vi "Settings Dialog.vi"(8 "error in (no error)":errorcluster, 11 "Settings in":T1) -> (0 "error out":errorcluster, 1 "Cancelled?":bool, 2 "UI Refresh Needed?":bool, 3 "Settings out":T1)   [LabVIEW 2018, in "Settings.lvlib"]
doc: "Dialog for selecting user specified settings."
uses:
  Settings.lvlib
  Settings.ctl
  Acquisition/Hardware Configuration.ctl
  Acquisition/Signal Type.ctl
  Logging/Logging Configuration.ctl
  TypeDef/Error LED.ctl
  <vilib>/Utility/xml.llb/Write to XML File(string).vi
  Acquisition/Acquisition.lvlib
  Logging/Logging.lvlib
panel:
  in  "Log File Path":path
  in  "Cancel Button":bool
  in  "OK Button":bool
  # "Non visible portion of dialog (needed for connector pane)."
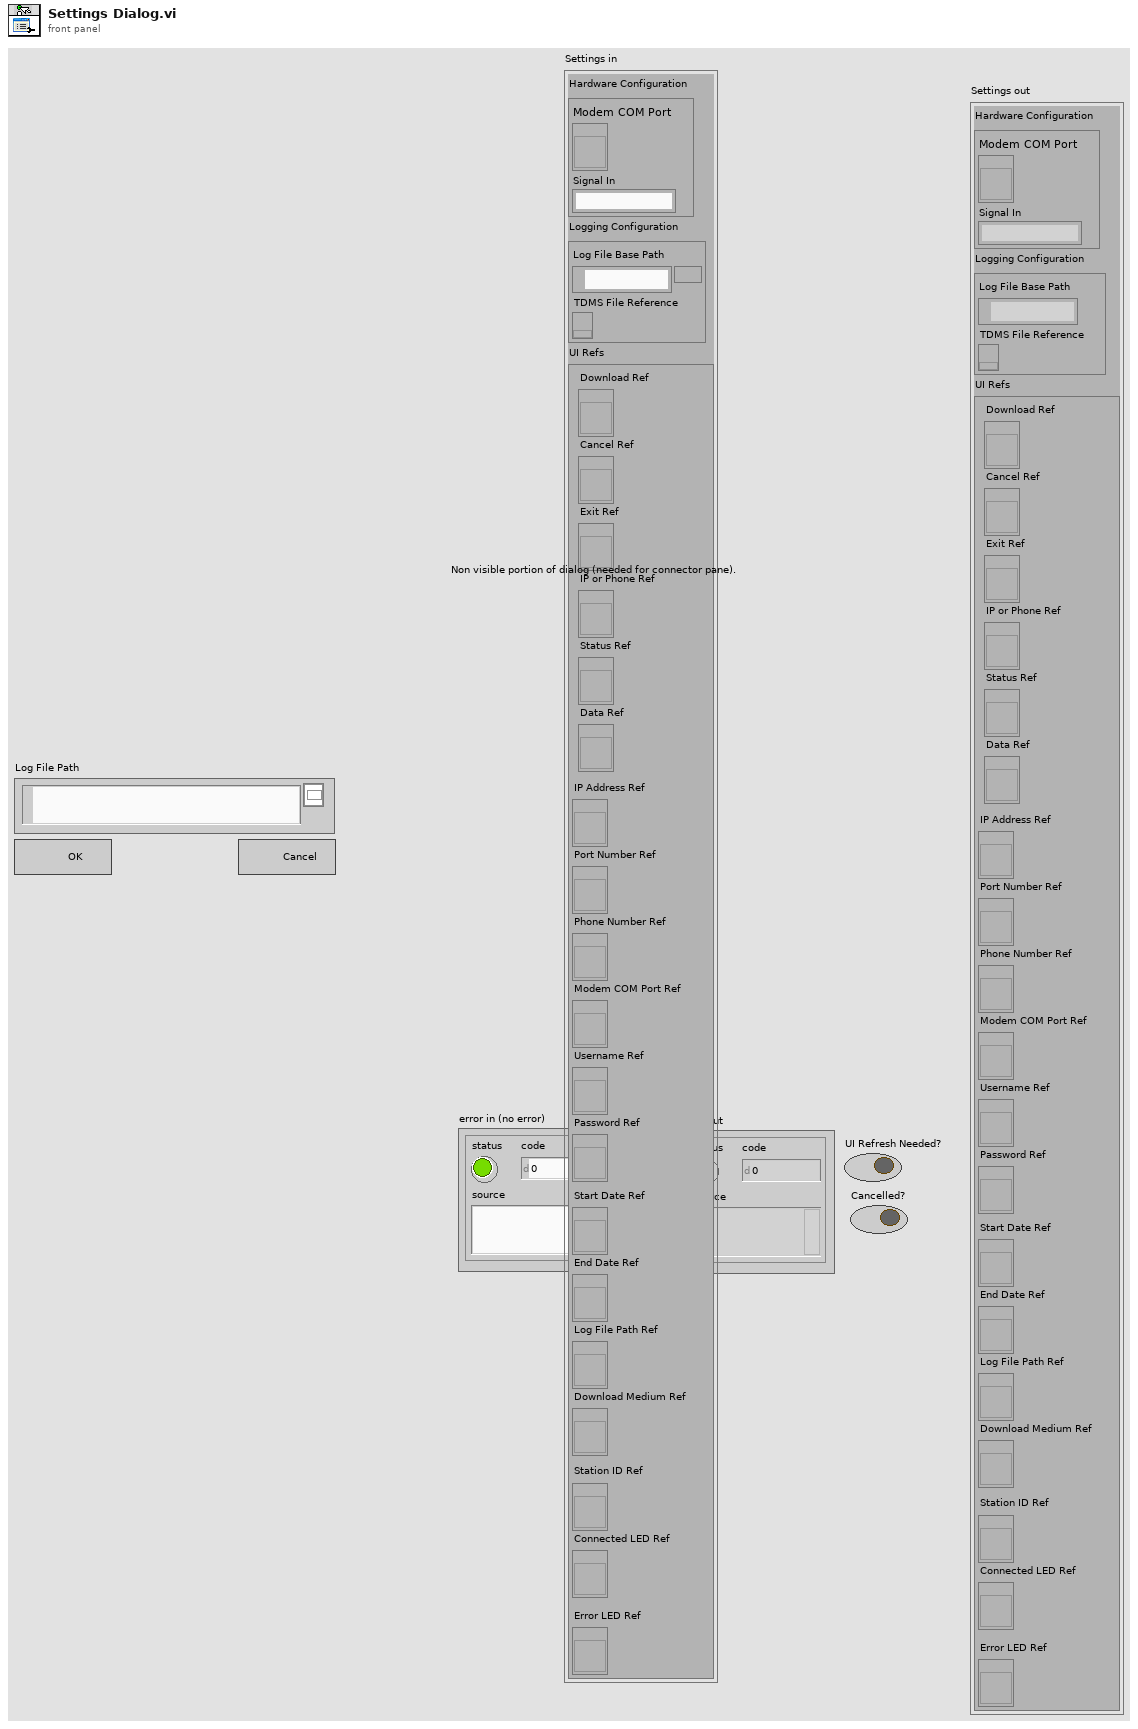
[diagram p1: front panel]
types:
  T1 = typedef "Settings.lvlib/Settings.ctl" = cluster{"Hardware Configuration":T2, "Logging Configuration":T4, "UI Refs":cluster{"Download Ref":refnum<vi>, "Cancel Ref":refnum<vi>, "Exit Ref":refnum<vi>, "IP or Phone Ref":refnum<vi>, "Status Ref":refnum<vi>, "Data Ref":refnum<vi>, "IP Address Ref":refnum<vi>, "Port Number Ref":refnum<vi>, "Phone Number Ref":refnum<vi>, "Modem COM Port Ref":refnum<vi>, "Username Ref":refnum<vi>, "Password Ref":refnum<vi>, "Start Date Ref":refnum<vi>, "End Date Ref":refnum<vi>, "Log File Path Ref":refnum<vi>, "Download Medium Ref":refnum<vi>, "Station ID Ref":refnum<vi>, "Connected LED Ref":refnum<vi>, "Error LED Ref":refnum<vi>}}
  T2 = typedef "Acquisition.lvlib/Hardware Configuration.ctl" = cluster{"Modem COM Port":refnum<vi>, "Signal In":T3}
  T3 = typedef "Acquisition.lvlib/Signal Type.ctl" = string
  T4 = typedef "Logging.lvlib/Logging Configuration.ctl" = cluster{"Log File Base Path":path, "TDMS File Reference":refnum<k34>}
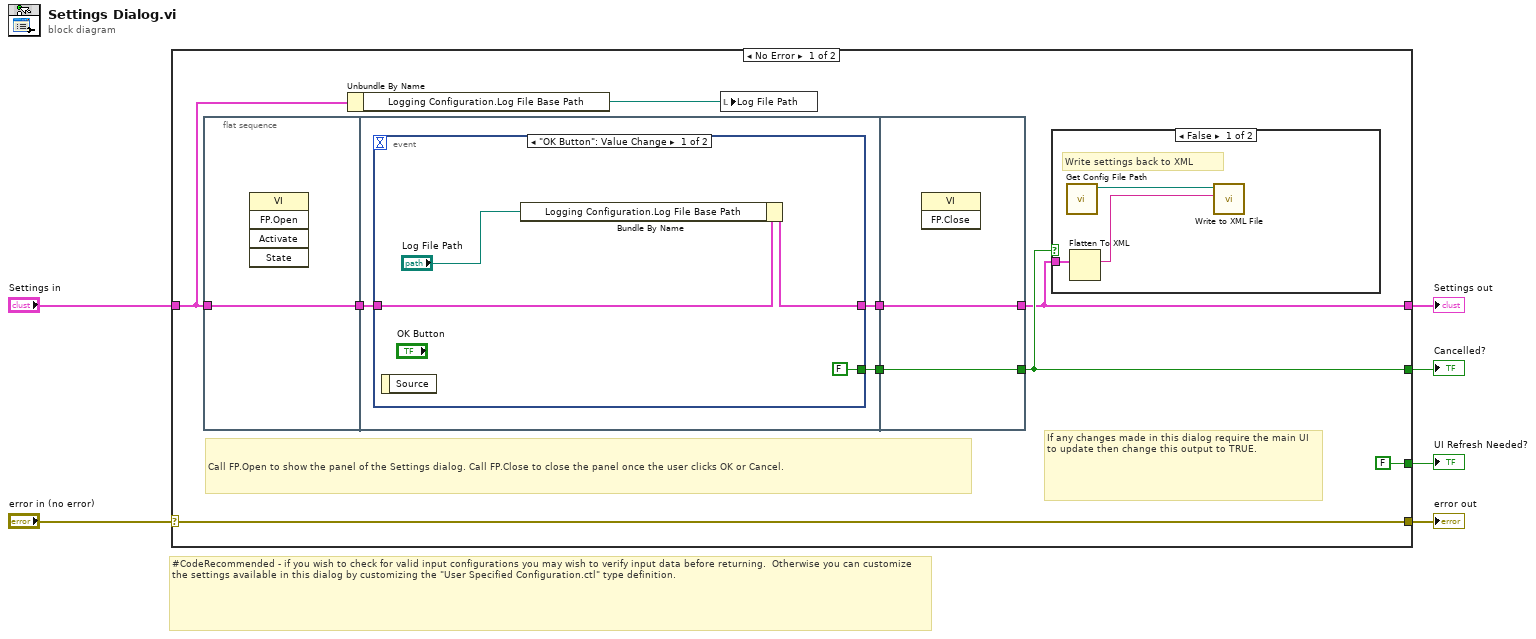
[diagram p0: block diagram]
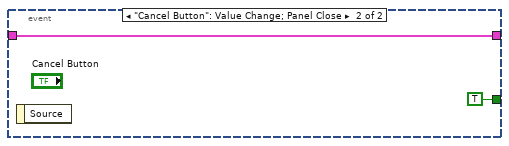
[diagram p2: hidden frame]
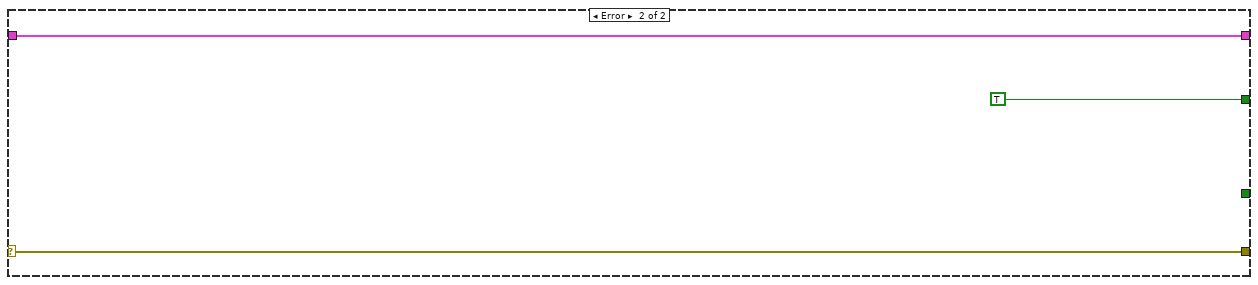
[diagram p4: hidden frame]
diagram:
  # "#CodeRecommended - if you wish to check for valid input configurations you may wish to verify input data before returning.  Otherwise you can customize the settings available in this dialog by customizing the \"User Specified Configuration.ctl\" type definition."
  n1 = case shown="No Error" "error in (no error)" {
    selector: "error in (no error)" -> [w15 w33]
    tunnel: [w15 w33] -> w5
    tunnel: "Settings in" -> [w11 w32]
    tunnel: [w12 w32] -> w3
    tunnel: [FALSE ("UI Refresh Needed?") _] -> w2
    tunnel: [w13 TRUE ("UI Refresh Needed?")] -> w1
    frame No Error {
      # "Call FP.Open to show the panel of the Settings dialog. Call FP.Close to close the panel once the user clicks OK or Cancel."
      # "If any changes made in this dialog require the main UI to update then change this output to TRUE."
      n2 = flat-sequence {
        tunnel: w11 -> [w16]
        tunnel: [w16] -> w9
        tunnel: w9 -> [w17]
        tunnel: [w19] -> w8
        tunnel: [w18] -> w7
        tunnel: [w26] -> w12
        tunnel: [w27] -> w13
        tunnel: w8 -> [w27]
        tunnel: w7 -> [w26]
        frame #0 {
          n3 = invoke class="VI" method="FP.Open"() -> ()  [unwired: 5 in, 5 out]
        }
        frame #1 {
          n4 = event shown="[0] \"OK Button\": Value Change" {
            selector: _ -> [_ _]
            dyn-events: _ -> [_ _]
            timeout: _ -> [_ _]
            tunnel: [w21 w25] -> w18
            tunnel: w17 -> [w22 w25]
            tunnel: [FALSE ("UI Refresh Needed?") TRUE ("UI Refresh Needed?")] -> w19
            event "OK Button": Value Change {
              n5 = event-data() -> ()  [unwired: 1 in, 1 out]
              n6 = Bundle By Name(cluster=w22, "Logging Configuration.Log File Base Path"="Log File Path") -> (w21:T1)
            }
            event "Cancel Button": Value Change; Panel Close {
              n7 = event-data() -> ()  [unwired: 1 in, 1 out]
            }
          }
        }
        frame #2 {
          n8 = invoke class="VI" method="FP.Close"() -> ()  [unwired: 3 in, 3 out]
        }
      }
      n9 = Unbundle By Name(w11) -> ("Logging Configuration.Log File Base Path"=w10:path)
      n10 = local write "Log File Path"(w10) -> ()
      n11 = case shown="False" w13 {
        tunnel: w12 -> [w29 _]
        frame False {
          # "Write settings back to XML"
          n12 = call "Get Config File Path.vi"() -> ("XML File Path"=w30:path)  [unwired: 10 in, 1 out]
          n13 = Flatten To XML(anything=w29) -> (xml string=w28:string)
          n14 = call-poly <vilib>:"Write to XML File.vi"("XML Input"=w28, "XML File Path"=w30) -> ()  [unwired: 7 in, 3 out]
        }
        frame True {
        }
      }
    }
    frame Error {
    }
  }
  "UI Refresh Needed?" <- w2
  "error out" <- w5
  "Settings out" <- w3
  "Cancelled?" <- w1
